vi "Calculate Waveform RMS average.vi"(8 "Error":errorcluster, 9 "Source Freq (HZ)":dbl, 11 "Buffer":T1) -> (0 "Error Out":errorcluster, 3 "Average Out":dbl)   [LabVIEW 2015]
uses:
  Universal Controls/Waveform_Data.ctl
  <vilib>/Analysis/baseanly.llb/Mean (DBL).vi
  <vilib>/Analysis/NI_AALBase.lvlib
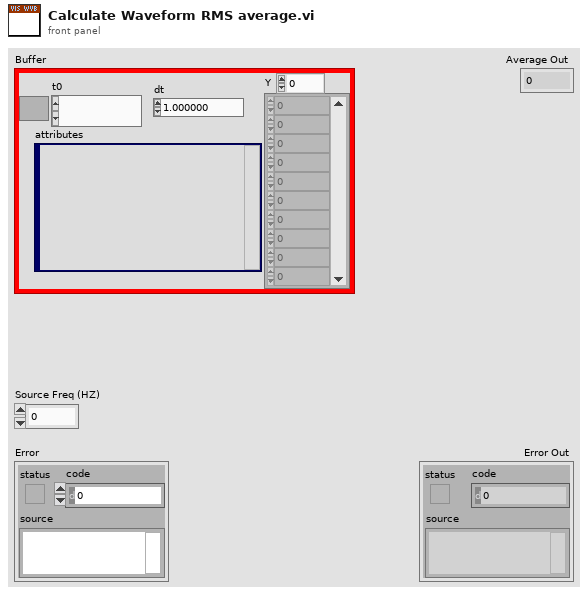
[diagram p1: front panel]
types:
  T1 = typedef "Waveform_Data.ctl" = waveform(dbl)
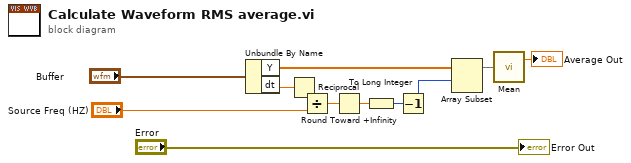
[diagram p0: block diagram]
diagram:
  n1 = Unbundle By Name("Buffer") -> ("Y"=w5:dbl[], "dt"=w7:dbl)
  n2 = Reciprocal(x=w7) -> (1/x=w11:dbl)
  n3 = Divide(x=w11, y="Source Freq (HZ)") -> (x/y=w9:dbl)
  n4 = Round Toward +Infinity(x=w9) -> (ceil(x): smallest int >= x=w10:dbl)
  n5 = To Long Integer(number=w10) -> (32bit integer=w2:i32)
  n6 = Decrement(x=w2) -> (x-1=w1:i32)
  n7 = Array Subset(array=w5, index=w1) -> (w8:dbl[])  [unwired: 1 in]
  n8 = call-poly <vilib>:"Mean.vi"("X"=w8) -> ("mean"=→"Average Out":dbl)  [unwired: 1 out]
  "Error Out" <- "Error"
